vi "search--unit test.vi"   [LabVIEW 2024, in "GUI.lvlib" / "Functions.lvlib"]
uses:
  Functions.lvlib
  <vilib>/addons/_JKI Toolkits/Caraya/classes/Assert/Assert Equal Value_Variant.vi
  <vilib>/addons/_JKI Toolkits/Caraya/classes/Test/Test.lvclass
  <vilib>/addons/_JKI Toolkits/Caraya/classes/Assert/Assert.lvclass
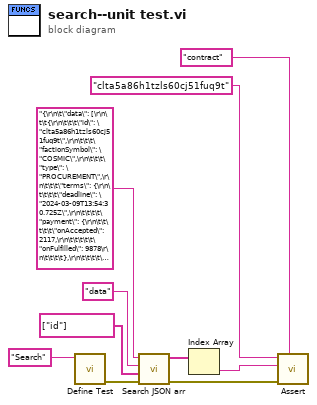
[diagram p0: block diagram]
diagram:
  n1 = call <vilib>:"Define Test.vi"("Label (VI Title)"="Search") -> ("error out"=w6:errorcluster)  [unwired: 9 in, 1 out]
  n2 = call "Search JSON arr.vi"("error in"=w6, "Search Terms"=string[] ["id"] ("Name Array 2"), "Name of arr"="data", "Response body"="{\r\n\t\"data\": [\r\n\t\t{\r\n\t\t\t\"id\": \"clta5a86h1tzls60cj51fuq9t\",\r\n\t\t\t\"factionSymbol\": \"COSMIC\",\r\n\t\t\t\"type\": \"PROCUREMENT\",\r\n\t\t\t\"terms\": {\r\n\t\t\t\t\"deadline\": \"2024-03-09T13:54:30.725Z\",\r\n\t\t\t\t\"payment\": {\r\n\t\t\t\t\t\"onAccepted\": 2117,\r\n\t\t\t\t\t\"onFulfilled\": 9878\r\n\t\t\t\t},\r\n\t\t\t\t\"deliver\": [\r\n\t\t\t\t\t{\r\n\t\t\t\t\t\t\"tradeSymbol\": \"COPPER_ORE\",\r\n\t\t\t\t\t\t\"destinationSymbol\": \"X1-JK49-H45\",\r\n\t\t\t\t\t\t\"unitsRequired\": 49,\r\n\t\t\t\t\t\t\"unitsFulfilled\": 0\r\n\t\t\t\t\t}\r\n\t\t\t\t]\r\n\t\t\t},\r\n\t\t\t\"accepted\": false,\r\n\t\t\t\"fulfilled\": false,\r\n\t\t\t\"expiration\": \"2024-03-03T13:54:30.725Z\",\r\n\t\t\t\"deadlineToAccept\": \"2024-03-03T13:54:30.725Z\"\r\n\t\t}\r\n\t],\r\n\t\"meta\": {\r\n\t\t\"total\": 1,\r\n\t\t\"page\": 1,\r\n\t\t\"limit\": 10\r\n\t}\r\n}") -> ("error out"=w5:errorcluster, "Respsonse"=w2:string[])  [unwired: 6 in]
  n3 = Index Array(array=w2) -> (element=w1:string)  [unwired: 1 in]
  n4 = call-poly <vilib>:"Assert.vi"("Label"="contract", "error in (no error)"=w5, "Y"=w1, "X"="clta5a86h1tzls60cj51fuq9t") -> ()  [unwired: 6 in, 2 out]
